vi "UI.vi"(8 "error in (no error)":errorcluster, 10 "subPanel":refnum<vi>, 11 "UI in":refnum<class "UI.lvclass">) -> (0 "error out":errorcluster, 3 "UI out":refnum<class "UI.lvclass">)   [LabVIEW 2018, in "UI.lvclass"]
doc: "Opens the UI Session. You need to pass a SubPanel Reference in order to make your embedded VIs show in it. This is the very first fuction you need to call."
uses:
  UI.lvclass
  UI.lvclass/UI.ctl
  setsubPanel.vi
  setEventReg.vi
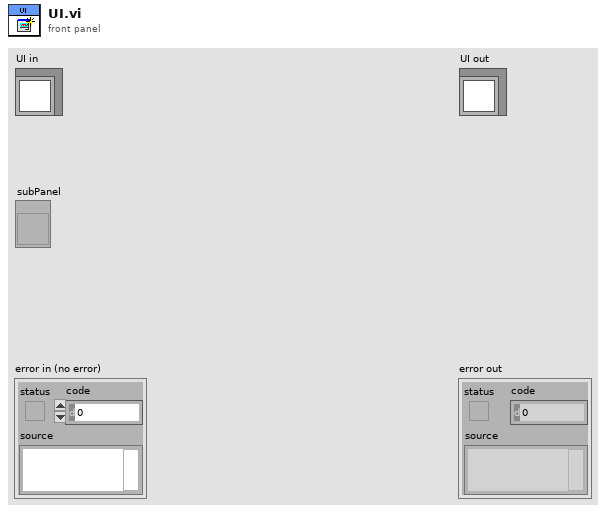
[diagram p1: front panel]
types:
  T1 = enum16{"Create", "Register", "Generate", "Unregister", "Destroy"}
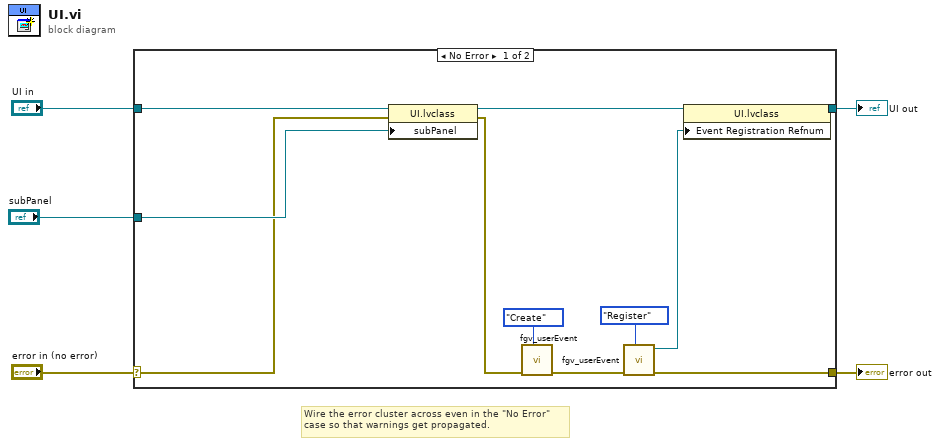
[diagram p0: block diagram]
diagram:
  # "Wire the error cluster across even in the \"No Error\"\ncase so that warnings get propagated."
  n1 = case shown="No Error" "error in (no error)" {
    selector: "error in (no error)" -> [w12 w18]
    tunnel: [w9 w18] -> w4
    tunnel: [w7 w17] -> w2
    tunnel: "UI in" -> [w16 w17]
    tunnel: "subPanel" -> [w14 _]
    frame No Error {
      n2 = property class="UI.lvclass"(reference=w16, error in=w12, "subPanel"=w14) -> (reference out=w15:refnum<class "UI.lvclass">, error out=w11:errorcluster)
      n3 = call "fgv_userEvent.vi"("Option"=T1."Create", "Error In"=w11) -> ("Error Out"=w13:errorcluster)  [unwired: 8 in, 1 out]
      n4 = call "fgv_userEvent.vi"("Option"=T1."Register", "Error In"=w13) -> ("Error Out"=w9:errorcluster, "Event Registration Refnum"=w6:refnum<event-registration>)  [unwired: 8 in]
      n5 = property class="UI.lvclass"(reference=w15, "Event Registration Refnum"=w6) -> (reference out=w7:refnum<class "UI.lvclass">)  [unwired: 1 in, 1 out]
    }
    frame Error {
    }
  }
  "error out" <- w4
  "UI out" <- w2
